vi "rystr_split_integers.vi"(0 "string":string, 1 "delimiter (',')":string=",") -> (6 "elements":i32[](array[numeric]))   [LabVIEW 2017]
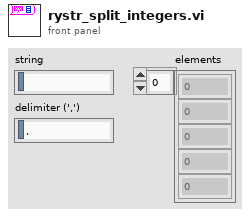
[diagram p1: front panel]
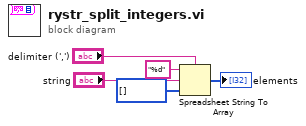
[diagram p0: block diagram]
diagram:
  n1 = Spreadsheet String To Array(delimiter (Tab)="delimiter (',')", format string="%d", spreadsheet string="string", array type (2D Dbl)=i32[] [] ("elements")) -> (array=→"elements":i32[])
